vi "CTR Start.vi"(8 "error in (no error)":errorcluster, 11 "Counter IO in":refnum<class "Counter IO.lvclass">) -> (0 "error out":errorcluster, 3 "Counter IO out":refnum<class "Counter IO.lvclass">)   [LabVIEW 2020, in "Instrument.lvlib" / "Counter IO.lvclass"]
uses:
  Counter IO.lvclass
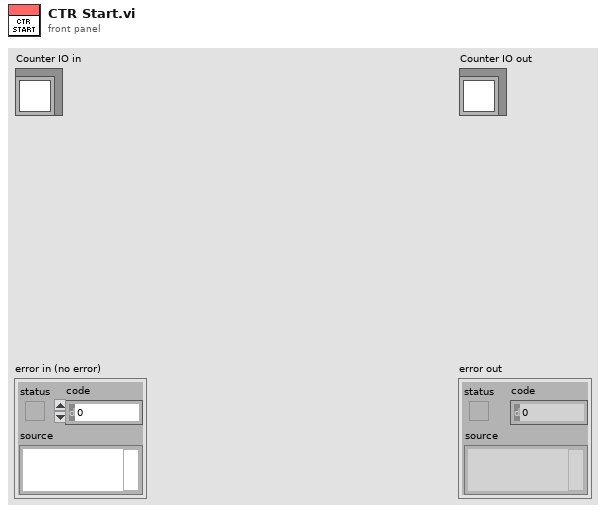
[diagram p1: front panel]
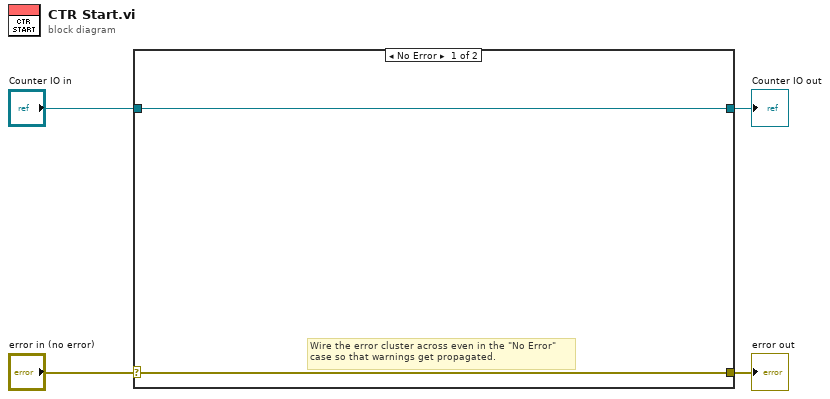
[diagram p0: block diagram]
diagram:
  n1 = case shown="No Error" "error in (no error)" {
    selector: "error in (no error)" -> [w5 w8]
    tunnel: [w5 w8] -> w3
    tunnel: [w6 w7] -> w1
    tunnel: "Counter IO in" -> [w6 w7]
    frame No Error {
      # "Wire the error cluster across even in the \"No Error\"\ncase so that warnings get propagated."
    }
    frame Error {
    }
  }
  "error out" <- w3
  "Counter IO out" <- w1
